vi "CreateIntegerArray.vi"() -> ()   [LabVIEW 2014]
uses:
  <vilib>/Analysis/1siggen.llb/Ramp Pattern by Samples.vi
  <vilib>/Analysis/NI_AALBase.lvlib
panel:
  in  "Minimum":dbl
  in  "Spacing":enum16{"Linear", "Logaraithmic"}(ring)
  out "Array":i8[](array[numeric])
  in  "Number of Elements":dbl
  in  "Maximum":dbl
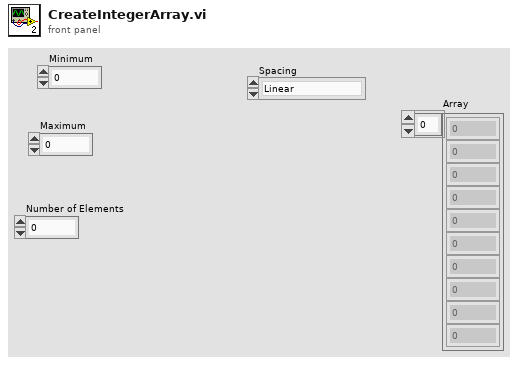
[diagram p1: front panel]
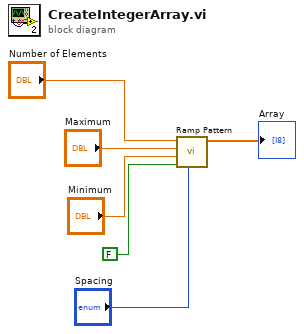
[diagram p0: block diagram]
diagram:
  n1 = call-poly <vilib>:"Ramp Pattern.vi"("type"="Spacing", "exclude end?"=FALSE, "start"="Minimum", "end"="Maximum", "samples"="Number of Elements") -> ("Ramp Pattern"=→"Array":dbl[])  [unwired: 5 in, 1 out]
